vi "UV-VIS GetHSSpeedSD.vi"(0 "Control in":refnum<class "CCD_camera.lvclass">, 1 "type":T1, 2 "index":i32, 3 "error in (no error)":errorcluster, 4 "channel":i32) -> (5 "Control out":refnum<class "CCD_camera.lvclass">, 6 "speed":sgl format="%.2f", 7 "DLL error code":u32, 8 "error out":errorcluster)   [LabVIEW 2020, in "CCD_camera.lvclass"]
doc: "As your AndorMCD[tm] system is capable of operating at more than one horizontal shift speed this function will return the actual speeds available. The value returned is in microseconds per pixel shift.\n\n<B>Parameters:</B>\nchannel - the AD channel\ntype - the horizontal read mode\n Valid values: 0 - speed of data readout\n 1 - speed of binning\n 2 - speed of dumping pixels\nindex - speed required\n Valid values: 0 to <B>GetNumberHSSpeeds</B>-1\nspeed - speed in micro-seconds per pixel shift\n\n<B>Error codes:</B>\nDRV_SUCCESS - Speed returned.\nDRV_NOT_INITIALIZED - System not initialized.\nDRV_ACQUIRING - Acquisition in progress.\nDRV_P1INVALID - Invalid channel.\nDRV_P2INVALID - Invalid horizontal read mode.\nDRV_P3INVALID - Invalid index."
uses:
  CCD_camera.lvclass
  atmcd32d.llb/HSSpeed_type typedef.ctl
  C:/dev/TRANCON/Classes/Detector/Detector.lvclass
  Detector.lvclass/Detector.ctl
  Detector.lvclass
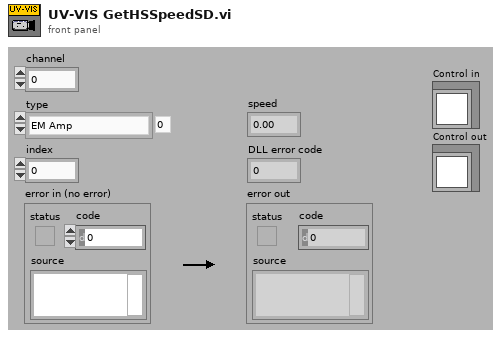
[diagram p1: front panel]
types:
  T1 = typedef "HSSpeed_type typedef.ctl" = enum16{"EM Amp", "Conventional Amp"}
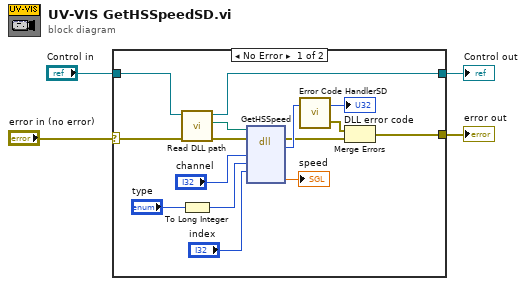
[diagram p0: block diagram]
diagram:
  n1 = case shown="No Error" "error in (no error)" {
    selector: "error in (no error)" -> [w11 w21]
    tunnel: [w6 w21] -> w3
    tunnel: [w5 w20] -> w2
    tunnel: "Control in" -> [w12 w20]
    frame No Error {
      n2 = call "Read DLL path.vi"("error in (no error)"=w11, "Detector in"=w12) -> ("error out"=w10:errorcluster, "DLL path"=w8:path, "Detector out"=w5:refnum<class "CCD_camera.lvclass">)  [unwired: 7 in]
      n3 = To Long Integer(number="type") -> (32bit integer=w15:i32)
      n4 = dll-call lib="S:/TRANCON/DLL/Atmcd32d.dll" fn="GetHSSpeed"(path in=w8, error in=w10, "channel"="channel", "type"=w15, "index"="index") -> (error out=w9:errorcluster, "return type"=w19:u32, "speed"=→"speed":sgl)  [unwired: 5 in, 1 out]
      n5 = call "Error Code HandlerSD.vi"("DLL error code"=w19) -> ("error out"=w7:errorcluster, "dup DLL error code"=→"DLL error code":u32)  [unwired: 1 in]
      n6 = Merge Errors(w7, w9) -> (w6:errorcluster)
    }
    frame Error {
    }
  }
  "error out" <- w3
  "Control out" <- w2
